vi "Write (1D U16).vi"(7 "count (-1: all)":i64=-1 format="%d elements", 8 "error in (no error)":errorcluster, 9 "offset (0)":u64 format="%d bytes", 10 "buffer in":u16[](array[numeric]), 11 "Pointer in":refnum<class "Pointer.lvclass">) -> (0 "error out":errorcluster, 1 "offset out":u64 format="%d bytes", 2 "buffer out":u16[](array[numeric]), 3 "Pointer out":refnum<class "Pointer.lvclass">)   [LabVIEW 2017, in "Memory Manager.lvlib" / "Pointer.lvclass"]
doc: "Writes <b>count</b> elements from the provided <b>buffer</b> to the address specified by <b>pointer + offset</b>.\n\n<b>Note:</b> This VI is <b>safe</b>.\n\nSafe means that this function evaluates the size parameter of <b>pointer</b> to ensure that is inbounds of allocated memory before peforming a memory read/write. Reading/writing more data to a pointer than it has allocated can corrupt or crash LabVIEW."
uses:
  Pointer.lvclass
  Pointer.lvclass/Pointer.ctl
  API/Accessors/Get Address.vi
  Protected/Errors.vi
  Protected/Error VIs/Null Pointer.vi
  Protected/Error VIs/Out of Bounds.vi
  API/Accessors/Get Size.vi
  Private/Count to Size.vi
  Protected/Error Building/Create Error.vi
  Protected/Error Building/Write Pointer Size.vi
  Protected/Error Building/Get Error Info.vi
  VIs/Write String into Source.vi
  VIs/Write Number into Source.vi
  VIs/VIs for Poly/Write U64 into Source.vi
  VIs/Set Error Source.vi
  VIs/Set Error Code.vi
  VIs/Set Error Status.vi
  Constants/Constants.vi
  Constants/Library Name.vi
  VIs/Create Error Cluster.vi
  VIs/VIs for Poly/Create Error Cluster (256B).vi
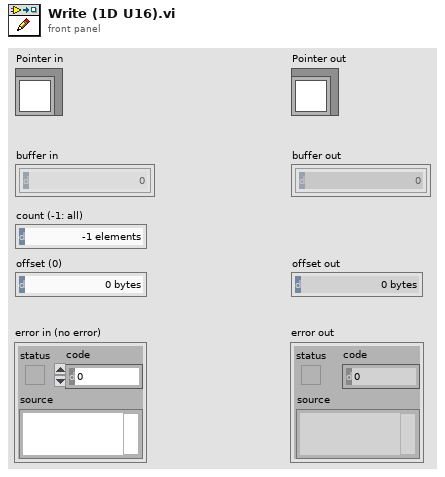
[diagram p1: front panel]
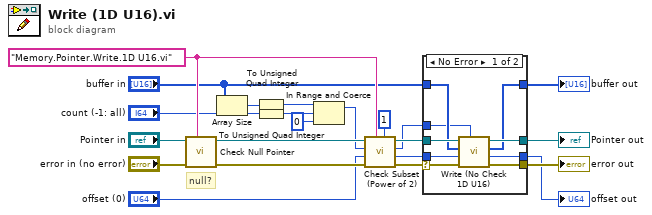
[diagram p0: block diagram]
diagram:
  w11 = "Memory.Pointer.Write.1D U16.vi" ("source vi name")
  # "null?"
  n1 = call "Check Null Pointer.vi"("source vi name"=w11, "error in (no error)"="error in (no error)", "Pointer in"="Pointer in") -> ("error out"=w13:errorcluster, "Pointer out"=w12:refnum<class "Pointer.lvclass">)  [unwired: 7 in]
  n2 = Array Size(array="buffer in") -> (size(s)=w10:i32)
  n3 = To Unsigned Quad Integer(1:w10) -> (0:w7:u64)
  n4 = To Unsigned Quad Integer(1:"count (-1: all)") -> (0:w8:u64)
  n5 = In Range and Coerce(upper limit=w7, x=w8, lower limit=u64 0) -> (coerced(x)=w5:u64)  [unwired: 1 out]
  n6 = call "Check Subset (Power of 2).vi"("power of 2"=i16 1, "source vi name"=w11, "error in (no error)"=w13, "offset (0)"="offset (0)", "count"=w5, "Pointer in"=w12) -> ("error out"=w22:errorcluster, "offset out"=w20:u64, "count"=w2:u64, "Pointer out"=w21:refnum<class "Pointer.lvclass">)  [unwired: 2 in]
  n7 = case shown="No Error" w22 {
    selector: w22 -> [w31 w34]
    tunnel: w21 -> [w29 w33]
    tunnel: w20 -> [w30 w35]
    tunnel: "buffer in" -> [w25 w32]
    tunnel: [w28 w34] -> w18
    tunnel: [w27 w33] -> w16
    tunnel: [w26 w35] -> w1
    tunnel: [w24 w32] -> w17
    tunnel: w2 -> [w23 _]
    frame No Error {
      n8 = call "Write (No Check 1D U16).vi"("count"=w23, "error in (no error)"=w31, "offset (0)"=w30, "buffer in"=w25, "Pointer in"=w29) -> ("error out"=w28:errorcluster, "offset out"=w26:u64, "buffer out"=w24:u16[], "Pointer out"=w27:refnum<class "Pointer.lvclass">)  [unwired: 3 in]
    }
    frame Error {
    }
  }
  "error out" <- w18
  "Pointer out" <- w16
  "buffer out" <- w17
  "offset out" <- w1
